vi "Open VI as Dialog.vi"(8 "error in (no error)":errorcluster, 10 "This Application":refnum<vi>, 11 "VI in":refnum<vi>) -> (0 "error out":errorcluster)   [LabVIEW 2013, in "Scan Engine editor node.lvclass"]
uses:
  Scan Engine editor node.lvclass
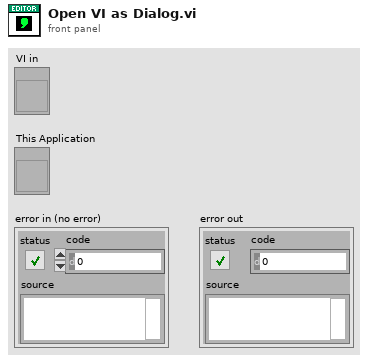
[diagram p1: front panel]
types:
  T1 = enum32{"Invalid", "Standard", "Closed", "Hidden", "Minimized", "Maximized"}
  T2 = enum32{"invalid app kind", "Development System", "Run Time System", "Student Edition", "Embedded LabVIEW", "Evaluation", "Custom"}
  T3 = enum32{"Invalid", "Default", "Floating", "Floating/Auto-Hide", "Modal"}
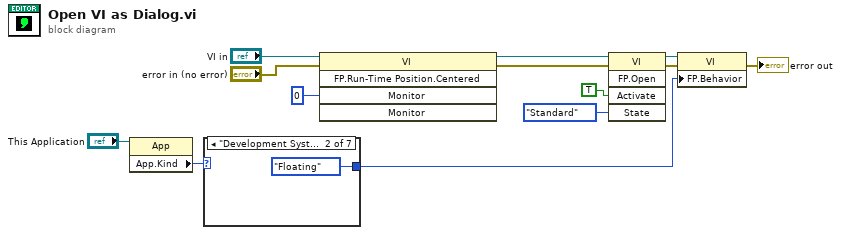
[diagram p0: block diagram]
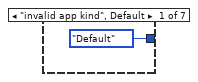
[diagram p2: hidden frame]
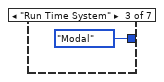
[diagram p3: hidden frame]
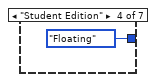
[diagram p4: hidden frame]
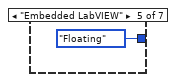
[diagram p5: hidden frame]
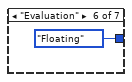
[diagram p6: hidden frame]
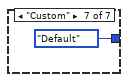
[diagram p7: hidden frame]
diagram:
  n1 = property class="App"(reference="This Application") -> ("App.Kind"=w7:T2)  [unwired: 1 in, 2 out]
  n2 = case shown="\"Development System\"" w7 {
    tunnel: [T3."Default" ("Front Panel Window:Behavior") T3."Floating" ("Front Panel Window:Behavior") T3."Modal" ("Front Panel Window:Behavior") T3."Floating" ("Front Panel Window:Behavior") T3."Floating" ("Front Panel Window:Behavior") T3."Floating" ("Front Panel Window:Behavior") T3."Default" ("Front Panel Window:Behavior")] -> w6
    frame "invalid app kind", Default {
    }
    frame "Development System" {
    }
    frame "Run Time System" {
    }
    frame "Student Edition" {
    }
    frame "Embedded LabVIEW" {
    }
    frame "Evaluation" {
    }
    frame "Custom" {
    }
  }
  n3 = invoke class="VI" method="FP.Run-Time Position.Centered"(reference="VI in", error in="error in (no error)", "Monitor"=i16 0) -> (reference out=w2:refnum<vi>, error out=w1:errorcluster)  [unwired: 2 in, 3 out]
  n4 = invoke class="VI" method="FP.Open"(reference=w2, error in=w1, "Activate"=TRUE ("Activate?"), "State"=T1."Standard") -> (reference out=w11:refnum<vi>, error out=w12:errorcluster)  [unwired: 1 in, 3 out]
  n5 = property class="VI"(reference=w11, error in=w12, "FP.Behavior"=w6) -> (error out=→"error out":errorcluster)  [unwired: 1 out]
